vi "Result.Append Name Prefix.vi"(7 "Append":bool, 9 "Name":string, 10 "Prefix":string) -> (1 "Name Out":string)   [LabVIEW 2019]
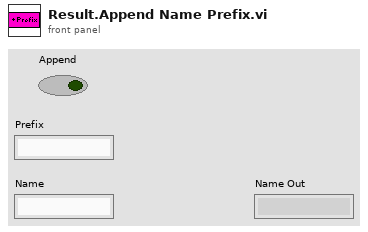
[diagram p1: front panel]
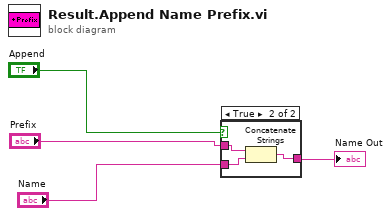
[diagram p0: block diagram]
diagram:
  n1 = case shown="True" "Append" {
    tunnel: "Name" -> [w5 w8]
    tunnel: [w5 w6] -> w4
    tunnel: "Prefix" -> [_ w7]
    frame False {
    }
    frame True {
      n2 = Concatenate Strings(w7, w8) -> (w6:string)
    }
  }
  "Name Out" <- w4
